vi "Populate Subpanels.vi"(8 "error in (no error)":errorcluster, 9 "View Labels (optional)":string[](array[string]), 10 "Views":refnum<class "Message Enqueuer.lvclass">[](array[class]), 11 "BoundViewManager In":refnum<class "BoundViewManager.lvclass">) -> (0 "error out":errorcluster, 3 "BoundViewManager Out":refnum<class "BoundViewManager.lvclass">)   [LabVIEW 2015, in "BoundViewManager.lvlib" / "BoundViewManager.lvclass"]
doc: "<License>\nCopyright © 2017 Composed Systems, LLC | All rights reserved\nwww.composed.io\n\nAuthor: Ethan Stern <ethan.stern@composed.io>\n\nThis software is provided \"AS IS\" WITHOUT WARRANTIES, either express or implied, AND IS FOR EDUCATIONAL PURPOSES ONLY.\n</License>"
uses:
  BoundViewManager.lvclass
  <vilib>/ActorFramework/Message Enqueuer/Message Enqueuer.lvclass
  BoundViewManager.lvclass/BoundViewManager.ctl
  Framework/IViewable/IViewable Messages/Insert View Msg/Insert View Msg.lvclass/Insert View Msg.ctl
  <vilib>/ActorFramework/Message Enqueuer/Message Enqueuer.lvclass/Message Enqueuer.ctl
  <vilib>/ActorFramework/Message Enqueuer/Enqueue.vi
  <vilib>/ActorFramework/Message Priority Queue/Priority Enqueue.vi
  Framework/IViewable/IViewable Messages/Insert View Msg/Insert View Msg.lvclass
  Framework/IViewManager/IViewManager/IViewManager.lvclass
  <vilib>/Composed Systems/Current Value Table/CurrentValueTable.lvclass
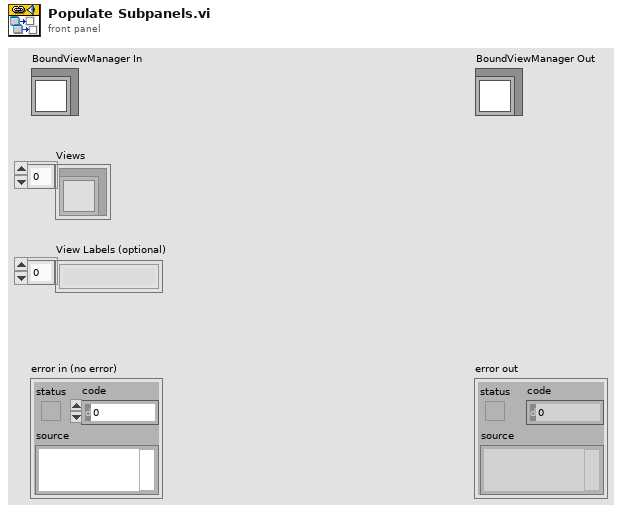
[diagram p1: front panel]
types:
  T1 = typedef "ProtectedSubpanel.lvlib/ProtectedSubpanel.lvclass/Protected Subpanel Reference.ctl" = refnum<data-value>
  T2 = typedef "CurrentValueTable.lvlib/CurrentValueTable.lvclass/CurrentValueTable Reference.ctl" = refnum<data-value>
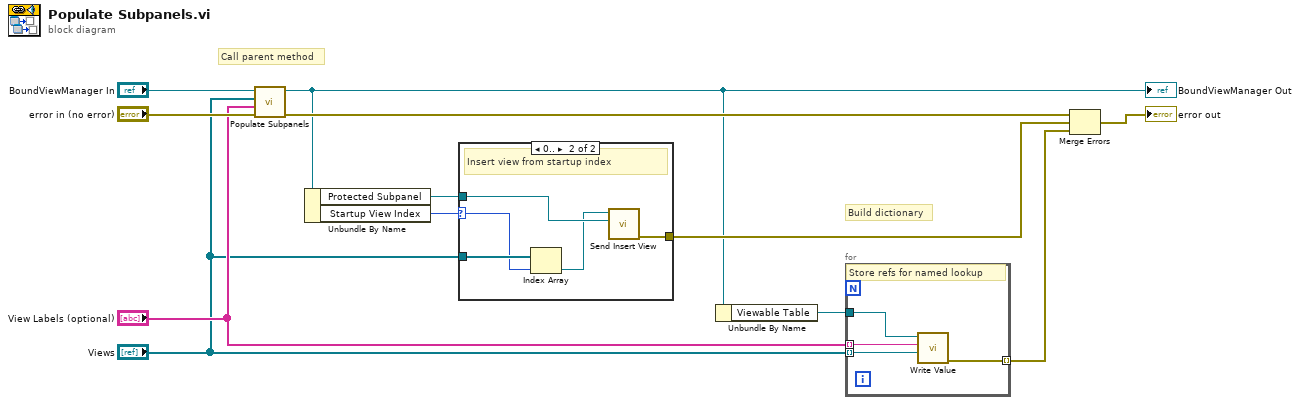
[diagram p0: block diagram]
diagram:
  # "Build dictionary"
  # "Call parent method"
  n1 = call-parent "Populate Subpanels.vi"("error in (no error)"="error in (no error)", "View Labels (optional)"="View Labels (optional)", "Views"="Views", "IViewManager In"="BoundViewManager In") -> ("error out"=w2:errorcluster, "IViewManager Out"=w1:refnum<class "BoundViewManager.lvclass">)  [unwired: 6 in]
  "BoundViewManager Out" <- w1
  n2 = Unbundle By Name(w1) -> ("Protected Subpanel"=w6:T1, "Startup View Index"=w4:i32)
  n3 = case shown="0.." w4 {
    selector: w4 -> [_ w14]
    tunnel: w6 -> [_ w17]
    tunnel: "Views" -> [_ w16]
    tunnel: [_ w13] -> w3
    frame ..-1 {
      # "No startup insert"
    }
    frame 0.. {
      # "Insert view from startup index"
      n4 = Index Array(array=w16, index=w14) -> (element=w15:refnum<class "Message Enqueuer.lvclass">)
      n5 = call "Send Insert View.vi"("Protected Subpanel"=w17, "Message Enqueuer"=w15) -> ("error out"=w13:errorcluster)  [unwired: 8 in, 1 out]
    }
  }
  n6 = Unbundle By Name(w1) -> ("Viewable Table"=w11:T2)
  n7 = for {
    tunnel: w11 -> [w21]
    tunnel: "View Labels (optional)" -> [w20] mode=indexing
    tunnel: "Views" -> [w19] mode=indexing
    tunnel: [w18] -> w7 mode=indexing
    # "Store refs for named lookup"
    n8 = call <vilib>:"Write Value.vi"("Value"=w19, "Data Name (Use Value Name)"=w20, "Current Value Table"=w21) -> ("error out"=w18:errorcluster)  [unwired: 7 in, 1 out]
  }
  n9 = Merge Errors(w2, w3, w7) -> (→"error out":errorcluster)
